vi "sched-check-compare.vi"(9 "sched-mode":enum16{"Hourly", "Daily", "Weekly", "Date"}(ring), 10 "sched-pairs":cluster{"start":T1, "stop":T1}[](array[cluster]) {"start" format="%<%H:%M %A>T"; "stop" format="%<%H:%M %d/%m/%y>T"}, 11 "time stamp":timestamp) -> (1 "Start":timestamp, 2 "Time":timestamp, 3 "Stop":timestamp, 4 "Found?":bool)   [LabVIEW 2024]
uses:
  <vilib>/Utility/miscctls.llb/LVDateTimeRec.ctl
  controls/UiScheduleTimestamp.ctl
panel:
  out "date time rec":T2
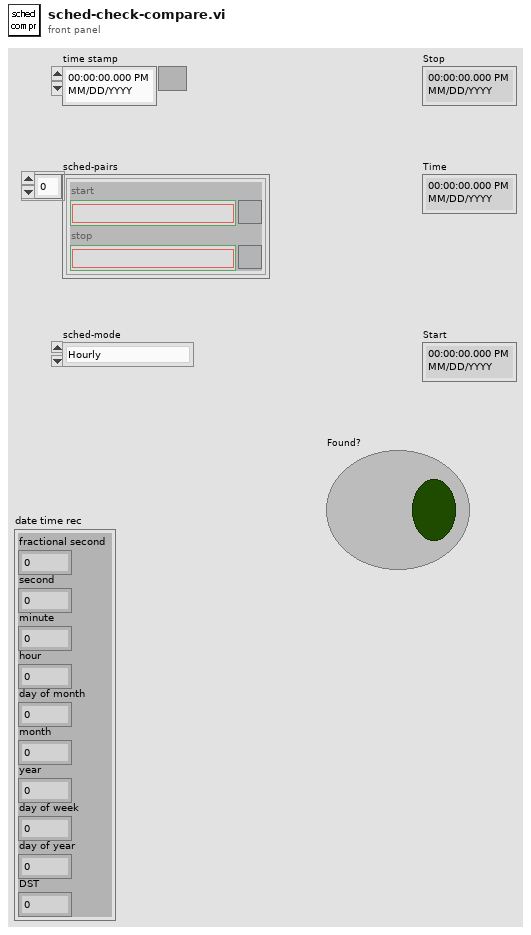
[diagram p1: front panel]
types:
  T1 = typedef "UiScheduleTimestamp.ctl" = timestamp
  T2 = typedef "LVDateTimeRec.ctl" = cluster{"fractional second":dbl, "second":i32, "minute":i32, "hour":i32, "day of month":i32, "month":i32, "year":i32, "day of week":i32, "day of year":i32, "DST":i32}
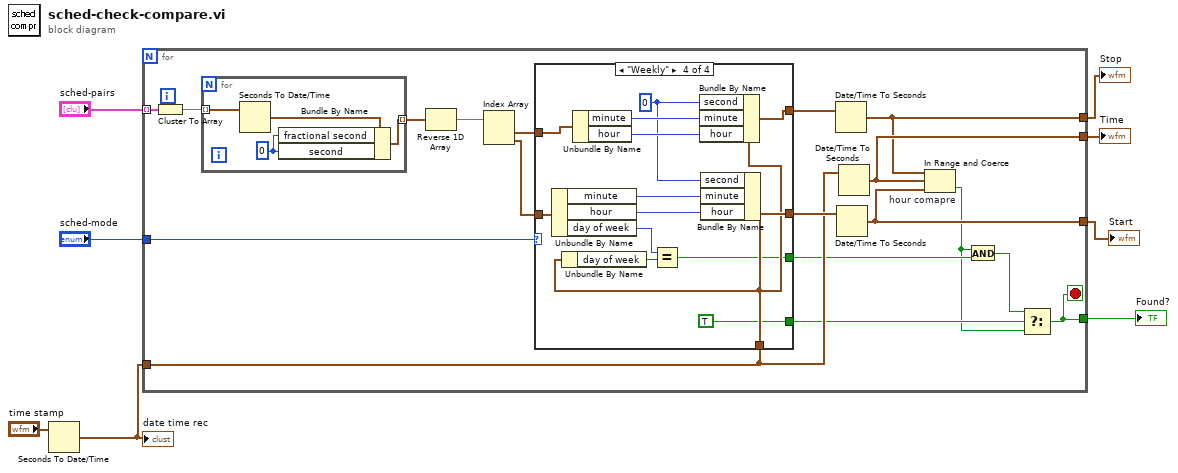
[diagram p0: block diagram]
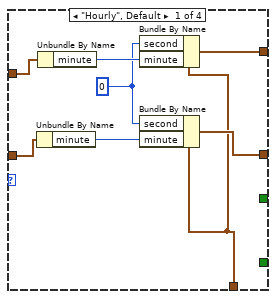
[diagram p2: hidden frame]
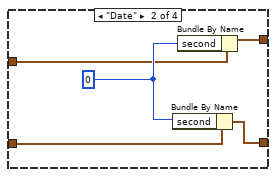
[diagram p3: hidden frame]
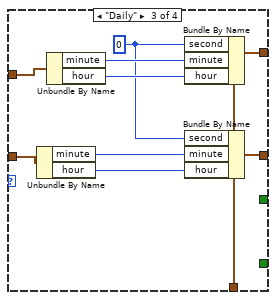
[diagram p4: hidden frame]
diagram:
  n1 = Seconds To Date/Time(time stamp (now)="time stamp") -> (date time rec=w2:T2)  [unwired: 1 in]
  "date time rec" <- w2
  n2 = for {
    tunnel: "sched-pairs" -> [w21] mode=indexing
    tunnel: [w9] -> w5
    tunnel: w2 -> [w24]
    tunnel: "sched-mode" -> [w23]
    tunnel: [w16] -> w6
    tunnel: [w15] -> w7
    tunnel: [w14] -> w8
    stop <- w9 stop-if-true
    n3 = Cluster To Array(cluster=w21) -> (array=w22:T1[])
    n4 = for {
      tunnel: w22 -> [w30] mode=indexing
      tunnel: [w27] -> w20 mode=indexing
      w28 = 0 ("second")
      n5 = Seconds To Date/Time(time stamp (now)=w30) -> (date time rec=w29:T2)  [unwired: 1 in]
      n6 = Bundle By Name(cluster=w29, "fractional second"=w28, "second"=w28) -> (w27:T2)
    }
    n7 = Reverse 1D Array(array=w20) -> (reversed array=w17:T2[])
    n8 = Index Array(array=w17) -> (element #1=w19:T2, element #2=w18:T2)  [unwired: 2 in]
    n9 = case shown="\"Weekly\"" w23 {
      tunnel: w19 -> [w38 w39 w53 w67]
      tunnel: w18 -> [w35 w41 w50 w64]
      tunnel: [w34 w40 w49 w63] -> w26
      tunnel: [w33 w42 w48 w62] -> w25
      tunnel: w24 -> [w32 _ w47 w58]
      tunnel: [_ _ _ w55] -> w13
      tunnel: [_ _ _ TRUE ("x = y?")] -> w12
      frame "Hourly", Default {
        w31 = 0 ("second")
        n10 = Unbundle By Name(w35) -> ("minute"=w36:i32)
        n11 = Unbundle By Name(w38) -> ("minute"=w37:i32)
        n12 = Bundle By Name(cluster=w32, "second"=w31, "minute"=w37) -> (w34:T2)
        n13 = Bundle By Name(cluster=w32, "second"=w31, "minute"=w36) -> (w33:T2)
      }
      frame "Date" {
        w43 = 0 ("second")
        n14 = Bundle By Name(cluster=w41, "second"=w43) -> (w42:T2)
        n15 = Bundle By Name(cluster=w39, "second"=w43) -> (w40:T2)
      }
      frame "Daily" {
        w44 = 0 ("second")
        n16 = Unbundle By Name(w50) -> ("minute"=w51:i32, "hour"=w45:i32)
        n17 = Unbundle By Name(w53) -> ("minute"=w52:i32, "hour"=w46:i32)
        n18 = Bundle By Name(cluster=w47, "second"=w44, "minute"=w52, "hour"=w46) -> (w49:T2)
        n19 = Bundle By Name(cluster=w47, "second"=w44, "minute"=w51, "hour"=w45) -> (w48:T2)
      }
      frame "Weekly" {
        w59 = 0 ("second")
        n20 = Unbundle By Name(w64) -> ("minute"=w65:i32, "hour"=w60:i32, "day of week"=w56:i32)
        n21 = Unbundle By Name(w58) -> ("day of week"=w57:i32)
        n22 = Unbundle By Name(w67) -> ("minute"=w66:i32, "hour"=w61:i32)
        n23 = Equal?(x=w56, y=w57) -> (x = y?=w55:bool)
        n24 = Bundle By Name(cluster=w58, "second"=w59, "minute"=w66, "hour"=w61) -> (w63:T2)
        n25 = Bundle By Name(cluster=w58, "second"=w59, "minute"=w65, "hour"=w60) -> (w62:T2)
      }
    }
    n26 = Date/Time To Seconds(2:w26) -> (0:w15:timestamp)  [unwired: 1 in]
    n27 = Date/Time To Seconds(2:w25) -> (0:w14:timestamp)  [unwired: 1 in]
    n28 = Date/Time To Seconds(2:w24) -> (0:w16:timestamp)  [unwired: 1 in]
    n29 = In Range and Coerce "hour comapre"(upper limit=w15, x=w16, lower limit=w14) -> (In Range?=w11:bool)  [unwired: 1 out]
    n30 = And(x=w11, y=w13) -> (x .and. y?=w10:bool)
    n31 = Select(t=w10, s=w12, f=w11) -> (s? t:f=w9:bool)
  }
  "Start" <- w8
  "Stop" <- w7
  "Time" <- w6
  "Found?" <- w5
